vi "Amp-sweep.vi"   [LabVIEW 2016]
uses:
  Global/Global Variables/global.vi
  Global/Global Variables/Data_Display_global.vi
  Instrument_Setup.vi
types:
  T1 = typedef "PSIO.ctl" = cluster{"Address":T2, "Version":enum16{"PS", "IPS"}}
  T2 = typedef "OxfordAddress.ctl" = cluster{"Com Port":i32, "ISOBUS Address":i32, "GPIB Address":i16, "Communication":enum16{"RS232", "ISOBUS", "GPIB", "Gateway"}}
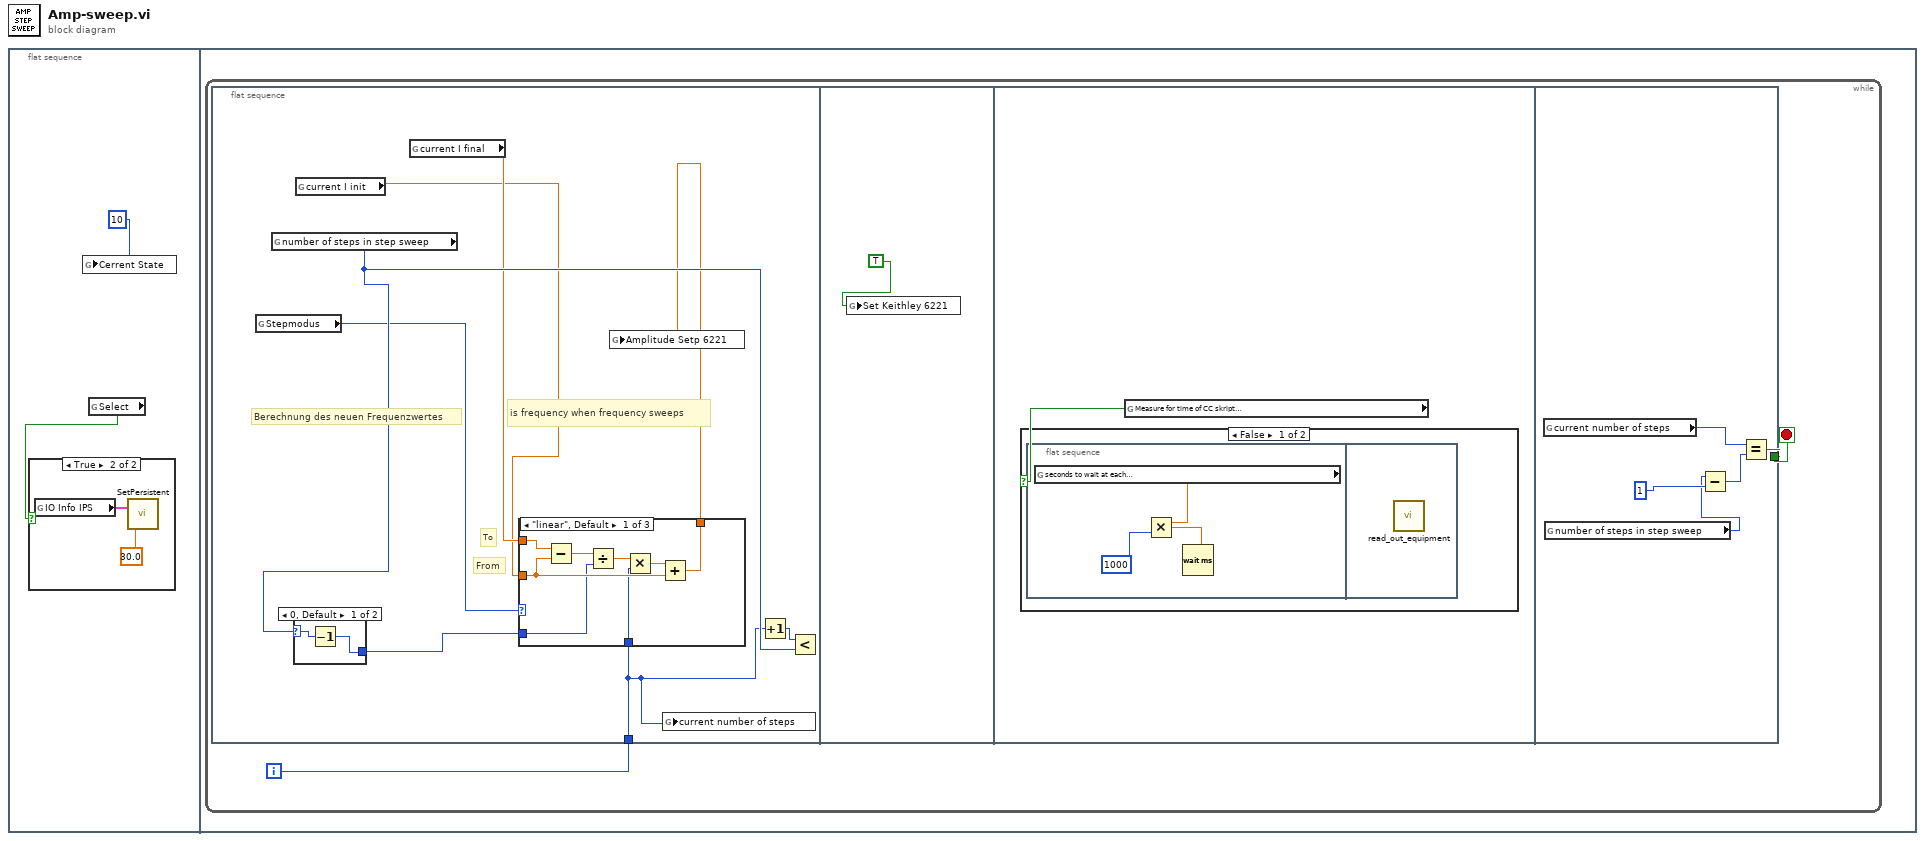
[diagram p0: block diagram]
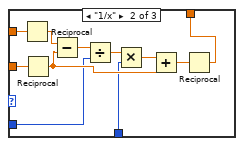
[diagram p4: hidden frame]
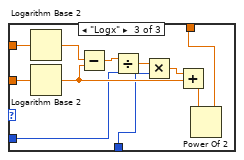
[diagram p5: hidden frame]
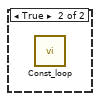
[diagram p6: hidden frame]
diagram:
  n1 = flat-sequence {
    frame #0 {
      n2 = global write "global.vi" "Cerrent State"(10) -> ()
      n3 = global read "Data_Display_global.vi" "Select"() -> (w1:bool)
      n4 = case shown="True" w1 {
        frame False {
        }
        frame True {
          n5 = global read "Instrument_Setup.vi" "IO Info IPS"() -> (w3:T1)
          n6 = call "SetPersistent.vi"("Switch Heater Dwell Time"=dbl[unit] 30.0, "IO Info"=w3) -> ()  [unwired: 1 in, 1 out]
        }
      }
    }
    frame #1 {
      n7 = while {
        i -> [w5]
        stop <- w6 stop-if-true
        n8 = flat-sequence {
          tunnel: w5 -> [w7]
          tunnel: [w56] -> w6
          frame #0 {
            # "From"
            # "To"
            # "is frequency when frequency sweeps"
            # "Berechnung des neuen Frequenzwertes"
            n9 = global read "Instrument_Setup.vi" "Stepmodus"() -> (w11:enum16{"linear", "1/x", "Logx"})
            n10 = global read "global.vi" "number of steps in step sweep"() -> (w12:i32)
            n11 = case shown="0, Default" w12 {
              selector: w12 -> [w16 w17]
              tunnel: [w15 w17] -> w13
              frame 0, Default {
                n12 = Decrement(x=w16) -> (x-1=w15:i32)
              }
              frame 1 {
              }
            }
            n13 = global read "global.vi" "current I init"() -> (w8:dbl)
            n14 = global read "global.vi" "current I final"() -> (w10:dbl)
            n15 = case shown="\"linear\", Default" w11 {
              tunnel: w10 -> [w25 w35 w47]
              tunnel: w8 -> [w22 w36 w46]
              tunnel: [w20 w30 w39] -> w9
              tunnel: w13 -> [w19 w27 w38]
              tunnel: w7 -> [w18 w26 w37]
              frame "linear", Default {
                n16 = Subtract(x=w25, y=w22) -> (x-y=w24:dbl)
                n17 = Divide(x=w24, y=w19) -> (x/y=w23:dbl)
                n18 = Multiply(x=w23, y=w18) -> (x*y=w21:dbl)
                n19 = Add(x=w21, y=w22) -> (x+y=w20:dbl)
              }
              frame "1/x" {
                n20 = Reciprocal(x=w35) -> (1/x=w29:dbl)
                n21 = Reciprocal(x=w36) -> (1/x=w28:dbl)
                n22 = Subtract(x=w29, y=w28) -> (x-y=w34:dbl)
                n23 = Divide(x=w34, y=w27) -> (x/y=w33:dbl)
                n24 = Multiply(x=w33, y=w26) -> (x*y=w32:dbl)
                n25 = Add(x=w32, y=w28) -> (x+y=w31:dbl)
                n26 = Reciprocal(x=w31) -> (1/x=w30:dbl)
              }
              frame "Logx" {
                n27 = Logarithm Base 2(1:w47) -> (0:w45:dbl)
                n28 = Logarithm Base 2(1:w46) -> (0:w41:dbl)
                n29 = Subtract(x=w45, y=w41) -> (x-y=w44:dbl)
                n30 = Divide(x=w44, y=w38) -> (x/y=w43:dbl)
                n31 = Multiply(x=w43, y=w37) -> (x*y=w42:dbl)
                n32 = Add(x=w42, y=w41) -> (x+y=w40:dbl)
                n33 = Power Of 2(x=w40) -> (2^x=w39:dbl)
              }
            }
            n34 = global write "Data_Display_global.vi" "Amplitude Setp 6221"(w9) -> ()
            n35 = global write "Data_Display_global.vi" "current number of steps"(w7) -> ()
            n36 = Increment(x=w7) -> (x+1=w14:i32)
            n37 = Less?(x=w14, y=w12) -> ()  [unwired: 1 out]
          }
          frame #1 {
            n38 = global write "Data_Display_global.vi" "Set Keithley 6221"(TRUE) -> ()
          }
          frame #2 {
            n39 = global read "Instrument_Setup.vi" "Measure for time of CC skript\nat each field step point"() -> (w49:bool)
            n40 = case shown="False" w49 {
              frame False {
                n41 = flat-sequence {
                  frame #0 {
                    n42 = global read "Instrument_Setup.vi" "seconds to wait at each\ncurrent step in a I-step sweep"() -> (w52:dbl)
                    n43 = Multiply(x=w52, y=u32 1000 ("milliseconds to wait")) -> (x*y=w50:dbl)
                    n44 = Wait (ms)(milliseconds to wait=w50) -> ()  [unwired: 1 out]
                  }
                  frame #1 {
                    n45 = call "read_out_equipment.vi"() -> ()  [unwired: 1 in]
                  }
                }
              }
              frame True {
                n46 = call "Const_loop.vi"() -> ()  [unwired: 4 in]
              }
            }
          }
          frame #3 {
            n47 = global read "Data_Display_global.vi" "current number of steps"() -> (w57:i32)
            n48 = global read "global.vi" "number of steps in step sweep"() -> (w54:i32)
            n49 = Subtract(x=w54, y=1) -> (x-y=w53:i32)
            n50 = Equal?(x=w57, y=w53) -> (x = y?=w56:bool)
          }
        }
      }
    }
  }
